vi "CheckShapeDescriptor.vi"(7 "Shape Type":T2(ring), 8 "error in (no error)":errorcluster, 10 "Descriptor Ref":refnum<vi>) -> (0 "error out":errorcluster, 2 "Descriptor":T1)   [LabVIEW 2015]
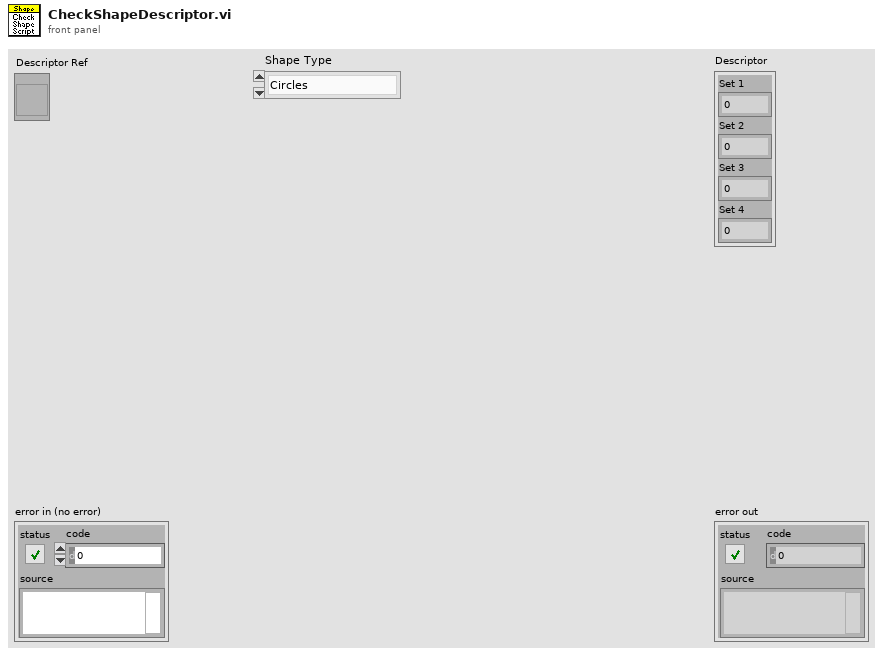
[diagram p1: front panel]
types:
  T1 = cluster{"Set 1":dbl, "Set 2":dbl, "Set 3":dbl, "Set 4":dbl}
  T2 = enum16{"Circles", "Ellipses", "Lines", "Rectangles"}
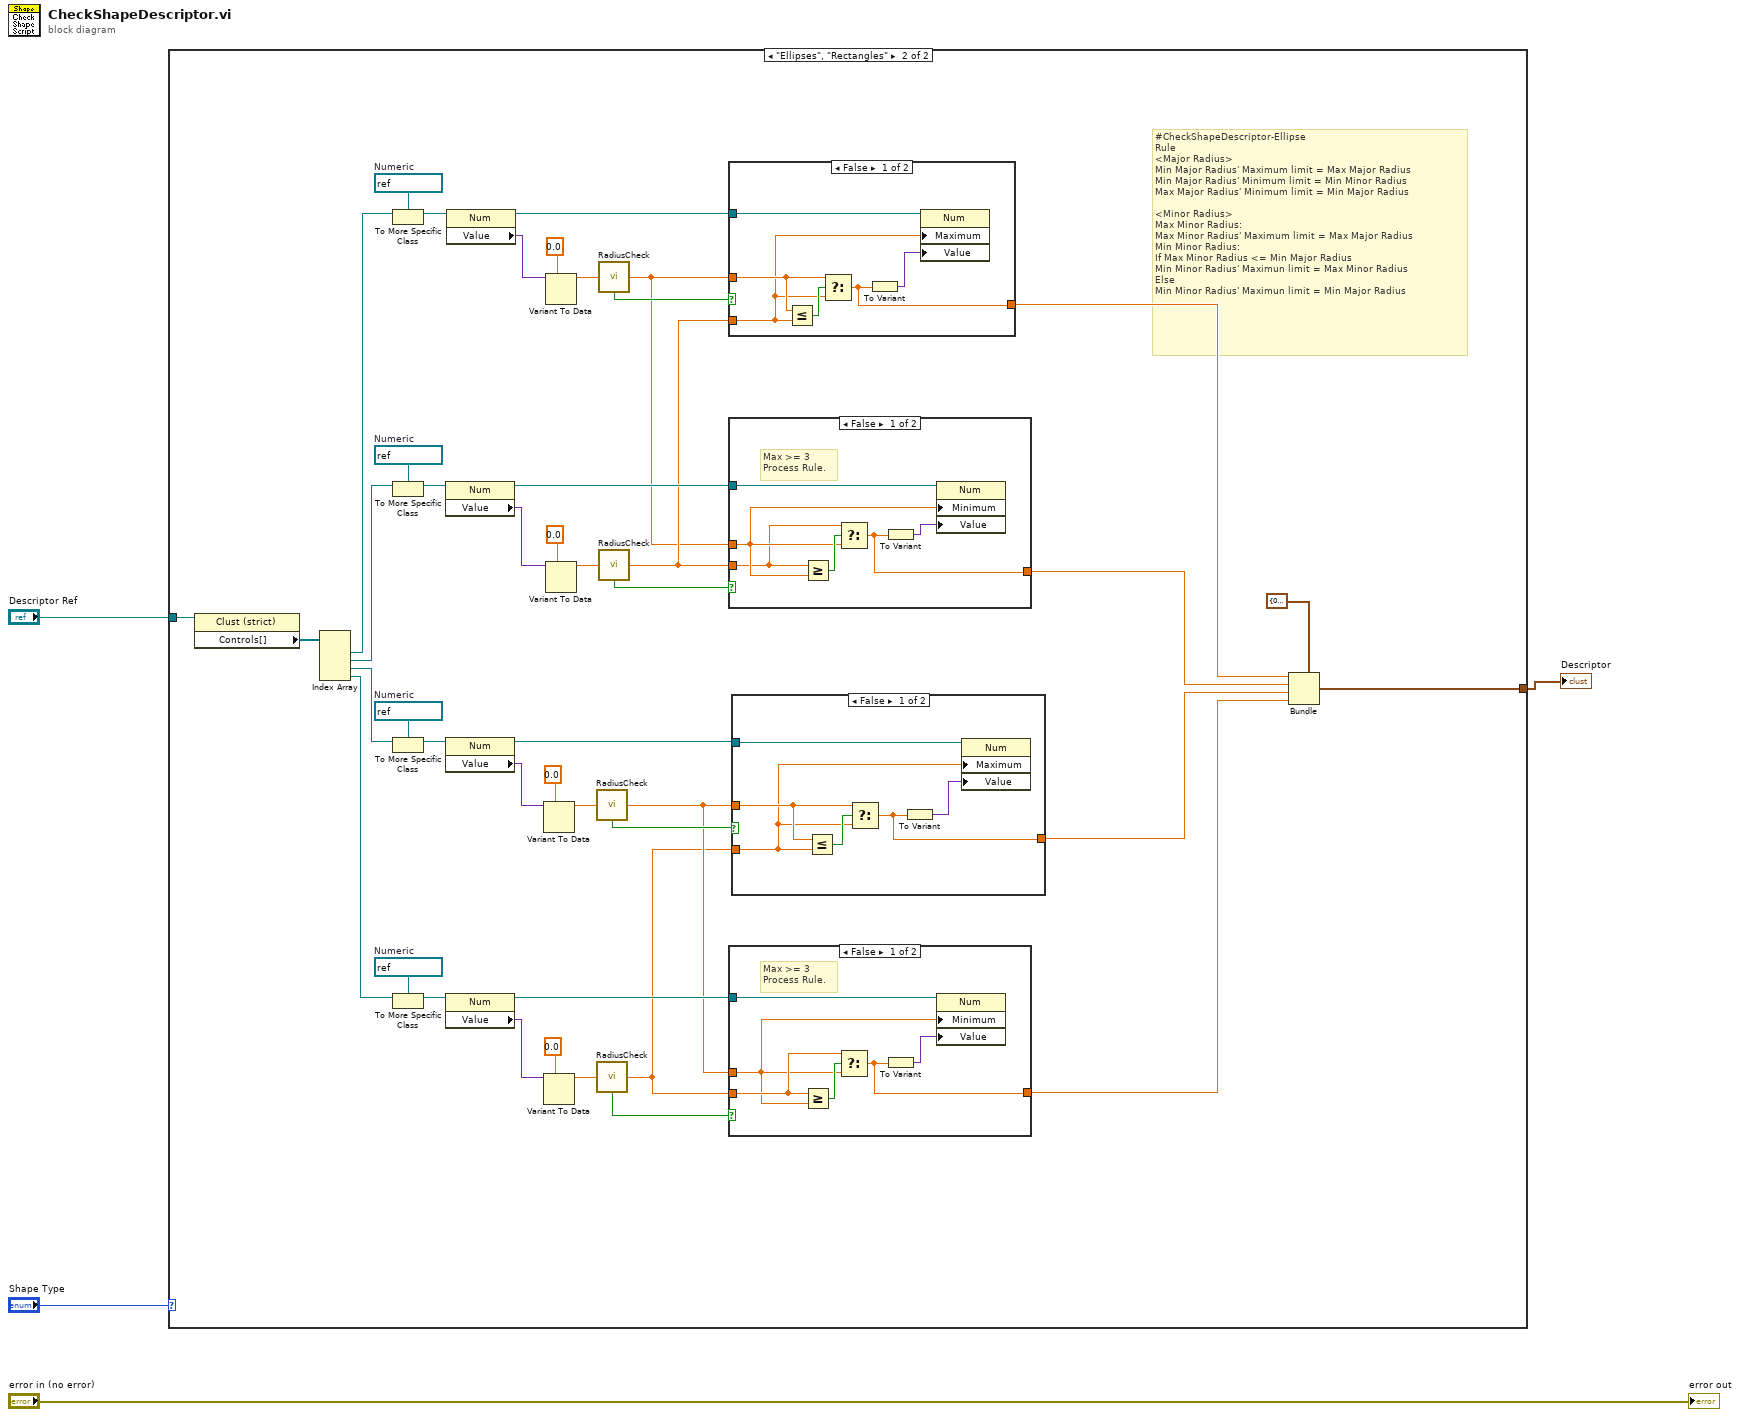
[diagram p0: block diagram]
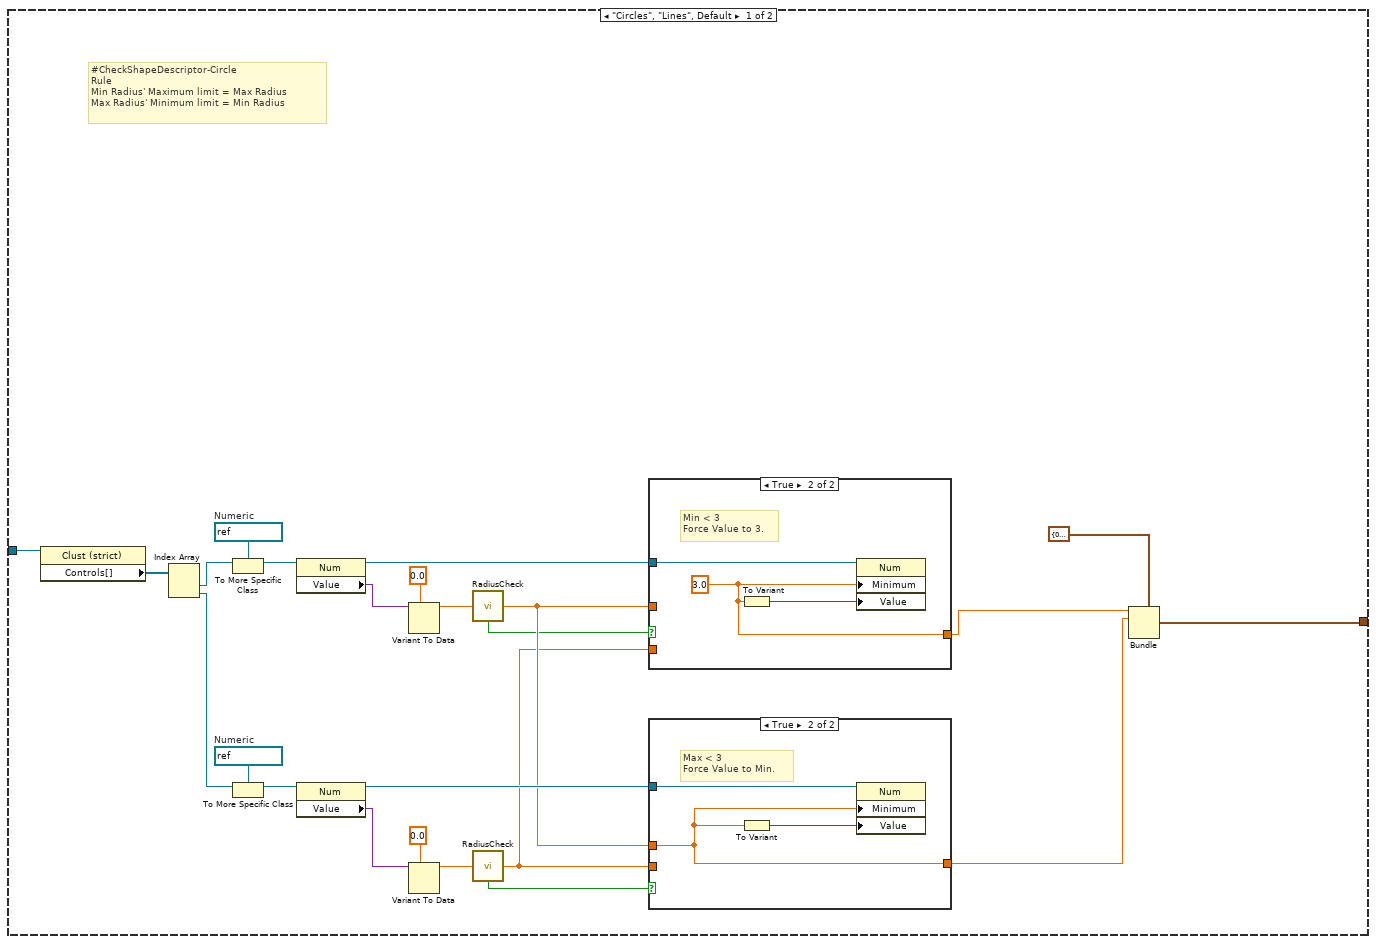
[diagram p2: hidden frame]
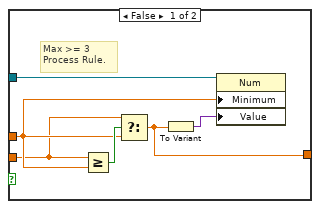
[diagram p3: hidden frame]
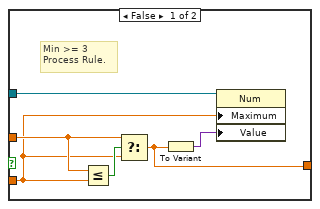
[diagram p4: hidden frame]
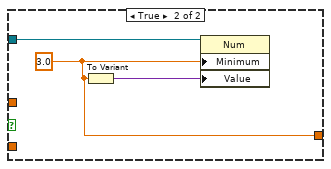
[diagram p5: hidden frame]
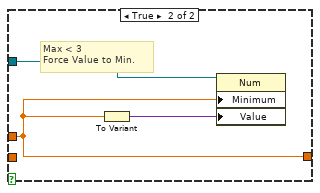
[diagram p6: hidden frame]
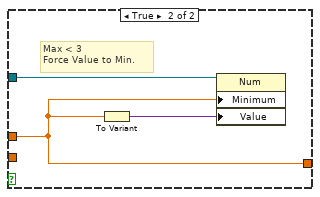
[diagram p7: hidden frame]
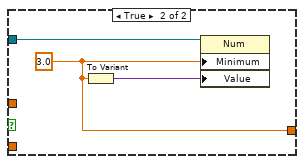
[diagram p8: hidden frame]
diagram:
  n1 = case shown="\"Ellipses\", \"Rectangles\"" "Shape Type" {
    tunnel: "Descriptor Ref" -> [w28 w89]
    tunnel: [w5 w56] -> w1
    frame "Circles", "Lines", Default {
      w22 = refnum<vi> refnum  # Numeric
      w26 = refnum<vi> refnum  # Numeric
      # "#CheckShapeDescriptor-Circle\nRule\nMin Radius' Maximum limit = Max Radius\nMax Radius' Minimum limit = Min Radius"
      n2 = property class="Clust (strict)"(reference=w28) -> ("Controls[]"=w27:refnum<vi>[])  [unwired: 1 in, 2 out]
      n3 = Index Array(array=w27) -> (element #1=w15:refnum<vi>, element #2=w21:refnum<vi>)  [unwired: 2 in]
      n4 = To More Specific Class(target class=w26, reference=w15) -> (specific class reference=w25:refnum<vi>)  [unwired: 1 in, 1 out]
      n5 = To More Specific Class(target class=w22, reference=w21) -> (specific class reference=w20:refnum<vi>)  [unwired: 1 in, 1 out]
      n6 = property class="Num"(reference=w25) -> (reference out=w16:refnum<vi>, "Value"=w24:variant)  [unwired: 1 in, 1 out]
      n7 = property class="Num"(reference=w20) -> (reference out=w17:refnum<vi>, "Value"=w18:variant)  [unwired: 1 in, 1 out]
      n8 = Variant To Data(type=0.0, Variant=w24) -> (data=w14:dbl)  [unwired: 1 in, 1 out]
      n9 = Variant To Data(type=0.0, Variant=w18) -> (data=w11:dbl)  [unwired: 1 in, 1 out]
      n10 = call "RadiusCheck.vi"("Radius In"=w14) -> ("Result"=w12:bool, "Radius Out"=w13:dbl)
      n11 = call "RadiusCheck.vi"("Radius In"=w11) -> ("Result"=w9:bool, "Radius Out"=w10:dbl)
      n12 = case shown="True" w12 {
        tunnel: w16 -> [w43 w46]
        tunnel: w13 -> [w40 _]
        tunnel: w10 -> [w39 _]
        tunnel: [w38 w44] -> w7
        frame False {
          # "Min >= 3\nProcess Rule."
          n13 = Less Or Equal?(x=w40, y=w39) -> (x <= y?=w42:bool)
          n14 = Select(t=w40, s=w42, f=w39) -> (s? t:f=w38:dbl)
          n15 = To Variant(anything=w38) -> (Variant=w41:variant)
          n16 = property class="Num"(reference=w43, "Maximum"=w39, "Value"=w41) -> ()  [unwired: 1 in, 2 out]
        }
        frame True {
          w44 = 3.0 ("Data Entry Limits:Minimum")
          # "Min < 3\nForce Value to 3."
          n17 = To Variant(anything=w44) -> (Variant=w45:variant)
          n18 = property class="Num"(reference=w46, "Minimum"=w44, "Value"=w45) -> ()  [unwired: 1 in, 2 out]
        }
      }
      n19 = case shown="True" w9 {
        tunnel: w17 -> [w34 w36]
        tunnel: w13 -> [w31 w35]
        tunnel: w10 -> [w30 _]
        tunnel: [w29 w35] -> w6
        frame False {
          # "Max >= 3\nProcess Rule."
          n20 = Greater Or Equal?(x=w30, y=w31) -> (x >= y?=w33:bool)
          n21 = Select(t=w30, s=w33, f=w31) -> (s? t:f=w29:dbl)
          n22 = To Variant(anything=w29) -> (Variant=w32:variant)
          n23 = property class="Num"(reference=w34, "Minimum"=w31, "Value"=w32) -> ()  [unwired: 1 in, 2 out]
        }
        frame True {
          # "Max < 3\nForce Value to Min."
          n24 = To Variant(anything=w35) -> (Variant=w37:variant)
          n25 = property class="Num"(reference=w36, "Minimum"=w35, "Value"=w37) -> ()  [unwired: 1 in, 2 out]
        }
      }
      n26 = Bundle(cluster=T1 {"Set 1"=0.0, "Set 2"=0.0, "Set 3"=0.0, "Set 4"=0.0} ("Descriptor"), "Set 1"=w7, "Set 2"=w6) -> (w5:T1)  [unwired: 2 in]
    }
    frame "Ellipses", "Rectangles" {
      w73 = refnum<vi> refnum  # Numeric
      w80 = refnum<vi> refnum  # Numeric
      w81 = refnum<vi> refnum  # Numeric
      w88 = refnum<vi> refnum  # Numeric
      # "#CheckShapeDescriptor-Ellipse\nRule\n<Major Radius>\nMin Major Radius' Maximum limit = Max Major Radius\nMin Major Radius' Minimum limit = Min Minor Radius\nMax Major Radius' Minimum limit = Min Major Radius\n\n<Minor Radius>\nMax Minor Radius:\nMax Minor Radius' Maximum limit = Max Major Radius\nMin Minor Radius:\nIf Max Minor Radius <= Min Major Radius\nMin Minor Radius' Maximun limit = Max Minor Radius\nElse\nMin Minor Radius' Maximun limit = Min Major Radius"
      n27 = property class="Clust (strict)"(reference=w89) -> ("Controls[]"=w90:refnum<vi>[])  [unwired: 1 in, 2 out]
      n28 = Index Array(array=w90) -> (element #1=w70:refnum<vi>, element #2=w69:refnum<vi>, element #3=w71:refnum<vi>, element #4=w72:refnum<vi>)  [unwired: 4 in]
      n29 = To More Specific Class(target class=w88, reference=w70) -> (specific class reference=w87:refnum<vi>)  [unwired: 1 in, 1 out]
      n30 = To More Specific Class(target class=w81, reference=w69) -> (specific class reference=w82:refnum<vi>)  [unwired: 1 in, 1 out]
      n31 = To More Specific Class(target class=w80, reference=w71) -> (specific class reference=w79:refnum<vi>)  [unwired: 1 in, 1 out]
      n32 = To More Specific Class(target class=w73, reference=w72) -> (specific class reference=w74:refnum<vi>)  [unwired: 1 in, 1 out]
      n33 = property class="Num"(reference=w82) -> (reference out=w62:refnum<vi>, "Value"=w83:variant)  [unwired: 1 in, 1 out]
      n34 = property class="Num"(reference=w79) -> (reference out=w52:refnum<vi>, "Value"=w78:variant)  [unwired: 1 in, 1 out]
      n35 = property class="Num"(reference=w74) -> (reference out=w61:refnum<vi>, "Value"=w75:variant)  [unwired: 1 in, 1 out]
      n36 = property class="Num"(reference=w87) -> (reference out=w64:refnum<vi>, "Value"=w86:variant)  [unwired: 1 in, 1 out]
      n37 = Variant To Data(type=0.0, Variant=w78) -> (data=w66:dbl)  [unwired: 1 in, 1 out]
      n38 = Variant To Data(type=0.0, Variant=w75) -> (data=w65:dbl)  [unwired: 1 in, 1 out]
      n39 = Variant To Data(type=0.0, Variant=w86) -> (data=w68:dbl)  [unwired: 1 in, 1 out]
      n40 = Variant To Data(type=0.0, Variant=w83) -> (data=w67:dbl)  [unwired: 1 in, 1 out]
      n41 = call "RadiusCheck.vi"("Radius In"=w66) -> ("Result"=w50:bool, "Radius Out"=w49:dbl)
      n42 = call "RadiusCheck.vi"("Radius In"=w65) -> ("Result"=w58:bool, "Radius Out"=w48:dbl)
      n43 = call "RadiusCheck.vi"("Radius In"=w68) -> ("Result"=w63:bool, "Radius Out"=w51:dbl)
      n44 = call "RadiusCheck.vi"("Radius In"=w67) -> ("Result"=w59:bool, "Radius Out"=w60:dbl)
      n45 = case shown="False" w63 {
        tunnel: w60 -> [w119 _]
        tunnel: w64 -> [w123 w125]
        tunnel: w51 -> [w122 _]
        tunnel: [w118 w124] -> w54
        frame False {
          n46 = Less Or Equal?(x=w122, y=w119) -> (x <= y?=w121:bool)
          n47 = Select(t=w122, s=w121, f=w119) -> (s? t:f=w118:dbl)
          n48 = To Variant(anything=w118) -> (Variant=w120:variant)
          n49 = property class="Num"(reference=w123, "Maximum"=w119, "Value"=w120) -> ()  [unwired: 1 in, 2 out]
        }
        frame True {
          w124 = 3.0 ("Data Entry Limits:Minimum")
          n50 = To Variant(anything=w124) -> (Variant=w126:variant)
          n51 = property class="Num"(reference=w125, "Minimum"=w124, "Value"=w126) -> ()  [unwired: 1 in, 2 out]
        }
      }
      n52 = case shown="False" w59 {
        tunnel: w62 -> [w114 w116]
        tunnel: w51 -> [w111 w115]
        tunnel: w60 -> [w110 _]
        tunnel: [w109 w115] -> w53
        frame False {
          # "Max >= 3\nProcess Rule."
          n53 = Greater Or Equal?(x=w110, y=w111) -> (x >= y?=w113:bool)
          n54 = Select(t=w110, s=w113, f=w111) -> (s? t:f=w109:dbl)
          n55 = To Variant(anything=w109) -> (Variant=w112:variant)
          n56 = property class="Num"(reference=w114, "Minimum"=w111, "Value"=w112) -> ()  [unwired: 1 in, 2 out]
        }
        frame True {
          # "Max < 3\nForce Value to Min."
          n57 = To Variant(anything=w115) -> (Variant=w117:variant)
          n58 = property class="Num"(reference=w116, "Minimum"=w115, "Value"=w117) -> ()  [unwired: 1 in, 2 out]
        }
      }
      n59 = case shown="False" w58 {
        tunnel: w61 -> [w105 w107]
        tunnel: w49 -> [w101 w106]
        tunnel: w48 -> [w102 _]
        tunnel: [w100 w106] -> w55
        frame False {
          # "Max >= 3\nProcess Rule."
          n60 = Greater Or Equal?(x=w102, y=w101) -> (x >= y?=w104:bool)
          n61 = Select(t=w102, s=w104, f=w101) -> (s? t:f=w100:dbl)
          n62 = To Variant(anything=w100) -> (Variant=w103:variant)
          n63 = property class="Num"(reference=w105, "Minimum"=w101, "Value"=w103) -> ()  [unwired: 1 in, 2 out]
        }
        frame True {
          # "Max < 3\nForce Value to Min."
          n64 = To Variant(anything=w106) -> (Variant=w108:variant)
          n65 = property class="Num"(reference=w107, "Minimum"=w106, "Value"=w108) -> ()  [unwired: 1 in, 2 out]
        }
      }
      n66 = case shown="False" w50 {
        tunnel: w48 -> [w92 _]
        tunnel: w52 -> [w91 w98]
        tunnel: w49 -> [w96 _]
        tunnel: [w95 w97] -> w47
        frame False {
          n67 = Less Or Equal?(x=w96, y=w92) -> (x <= y?=w94:bool)
          n68 = Select(t=w96, s=w94, f=w92) -> (s? t:f=w95:dbl)
          n69 = To Variant(anything=w95) -> (Variant=w93:variant)
          n70 = property class="Num"(reference=w91, "Maximum"=w92, "Value"=w93) -> ()  [unwired: 1 in, 2 out]
        }
        frame True {
          w97 = 3.0 ("Data Entry Limits:Minimum")
          n71 = To Variant(anything=w97) -> (Variant=w99:variant)
          n72 = property class="Num"(reference=w98, "Minimum"=w97, "Value"=w99) -> ()  [unwired: 1 in, 2 out]
        }
      }
      n73 = Bundle(cluster=T1 {"Set 1"=0.0, "Set 2"=0.0, "Set 3"=0.0, "Set 4"=0.0} ("Descriptor"), "Set 1"=w54, "Set 2"=w53, "Set 3"=w47, "Set 4"=w55) -> (w56:T1)
    }
  }
  "Descriptor" <- w1
  "error out" <- "error in (no error)"
